vi "VCS Get Interface Name Selection.vi"(8 "error in (no error)":errorcluster, 10 "startOfSelection in":i32, 11 "device in":T1={"deviceName"="EPOS2", "protocolStackName"="MAXON SERIAL V2", "interfaceName"="", "portName"=""}) -> (0 "error out":errorcluster, 1 "interfaceNameSel out":string, 2 "endOfSelection out":i32, 3 "device out":T1={"deviceName"="EPOS2", "protocolStackName"="", "interfaceName"="", "portName"=""})   [LabVIEW 2010]
doc: "<B>VCS Get Interface Name Selection</B> returns all available interface names."
uses:
  Resources/EposCmd.dll
  Resources/EposCmd64.dll
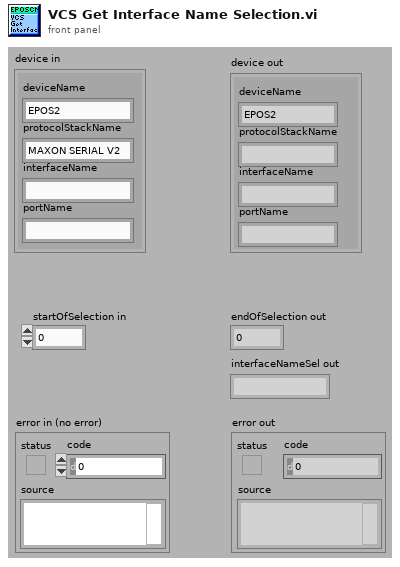
[diagram p1: front panel]
types:
  T1 = cluster{"deviceName":string, "protocolStackName":string, "interfaceName":string, "portName":string}
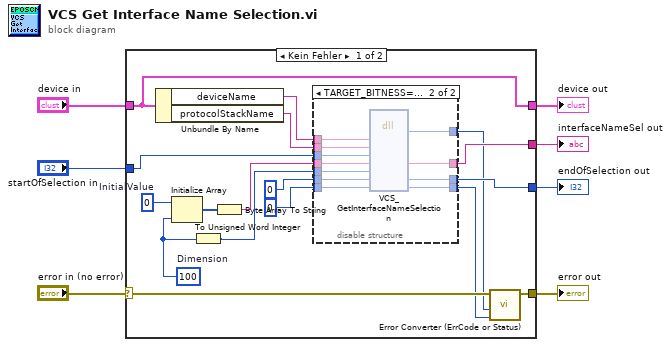
[diagram p0: block diagram]
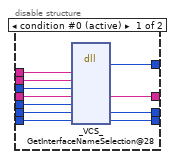
[diagram p2: hidden frame]
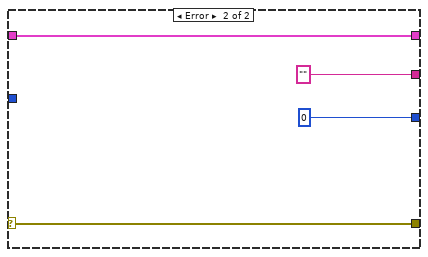
[diagram p3: hidden frame]
diagram:
  n1 = case shown="Kein Fehler" "error in (no error)" {
    selector: "error in (no error)" -> [w22 w50]
    tunnel: [w21 w50] -> w6
    tunnel: "startOfSelection in" -> [w24 _]
    tunnel: [w17 "" ("pInterfaceNameSel")] -> w4
    tunnel: [w23 0 ("pEndOfSelection")] -> w3
    tunnel: "device in" -> [w11 w49]
    tunnel: [w11 w49] -> w1
    frame No Error {
      w15 = u8 0  # InitialValue
      w8 = 100  # Dimension
      n2 = Unbundle By Name(w11) -> ("deviceName"=w19:string, "protocolStackName"=w18:string)
      n3 = Initialize Array(w15, w8) -> (w16:u8[])
      n4 = To Unsigned Word Integer(number=w8) -> (unsigned 16bit integer=w9:u16)
      n5 = Byte Array To String(unsigned byte array=w16) -> (string=w14:string)
      n6 = disable-structure shown="TARGET_BITNESS==64" {
        disable-tunnel: w24 -> [w35 w46]
        disable-tunnel: [w34 w45] -> w23
        disable-tunnel: [w33 w44] -> w20
        disable-tunnel: w19 -> [w32 w43]
        disable-tunnel: w18 -> [w31 w42]
        disable-tunnel: [w30 w41] -> w17
        disable-tunnel: w14 -> [w29 w40]
        disable-tunnel: 0 ("pEndOfSelection") -> [w28 w39]
        disable-tunnel: u32 0 ("pErrorCode") -> [w27 w38]
        disable-tunnel: [w26 w37] -> w10
        disable-tunnel: w9 -> [w25 w36]
        frame condition #0 (active) {
          n7 = dll-call lib="C:/Sources/LabView/maxon EPOS/Resources/EposCmd.*" fn="_VCS_GetInterfaceNameSelection@28"("DeviceName"=w32, "ProtocolStackName"=w31, "StartOfSelection"=w35, "pInterfaceNameSel"=w29, "MaxStrSize"=w25, "pEndOfSelection"=w28, "pErrorCode"=w27) -> (w26:i32, "pInterfaceNameSel"=w30:string, "pEndOfSelection"=w34:i32, "pErrorCode"=w33:u32)  [unwired: 7 in, 2 out]
        }
        frame condition #1 {
          n8 = dll-call lib="C:/setup/Resources/EposCmd64.*" fn="VCS_GetInterfaceNameSelection" ("EposCmd.dll:_VCS_GetInterfaceNameSelection@28")("DeviceName"=w43, "ProtocolStackName"=w42, "StartOfSelection"=w46, "pInterfaceNameSel"=w40, "MaxStrSize"=w36, "pEndOfSelection"=w39, "pErrorCode"=w38) -> ("Rückgabetyp"=w37:i32, "pInterfaceNameSel"=w41:string, "pEndOfSelection"=w45:i32, "pErrorCode"=w44:u32)  [unwired: 7 in, 2 out]
        }
      }
      n9 = call "Error Converter (ErrCode or Status).vi"("error code"=w20, "return type"=w10, "error in (no error)"=w22) -> ("error out"=w21:errorcluster)  [unwired: 7 in]
    }
    frame Error {
    }
  }
  "interfaceNameSel out" <- w4
  "endOfSelection out" <- w3
  "error out" <- w6
  "device out" <- w1
